vi "Change Unit.vi"(0 "Rigol DG822 Sine in":refnum<class "Rigol DG822 Sine.lvclass">, 9 "ParamTags":T1, 11 "error in (no error)":errorcluster, 12 "New Value":u16, 14 "Old Value":u16) -> (4 "Rigol DG822 Sine out":refnum<class "Rigol DG822 Sine.lvclass">, 15 "error out":errorcluster)   [LabVIEW 2021, in "Rigol DG822 UI.lvlib" / "Rigol DG822 Sine.lvlib" / "Rigol DG822 Sine.lvclass"]
uses:
  Rigol DG822 Sine.lvclass
  Rigol DG822 UI/lib/controls.llb/WaveformParamTags.ctl
  Rigol DG822 UI/lib/controls.llb/FreqUnit.ctl
  Rigol DG822 Sine.lvclass/Rigol DG822 Sine.ctl
  Rigol DG822 UI/lib/controls.llb/PeriodUnit.ctl
  Rigol DG822 UI/lib/controls.llb/AmplUnit.ctl
  Rigol DG822 UI/lib/controls.llb/HighLUnit.ctl
  Rigol DG822 UI/lib/controls.llb/OffsetUnit.ctl
  Rigol DG822 UI/lib/controls.llb/LowLUnit.ctl
  General/Files/lvlibp/Actors.lvlibp/Actors/Actors/Actors.lvclass
  D:/LabVIEW/General/Files/lvlibp/Actors.lvlibp/Actors/Actors/Actors.lvclass
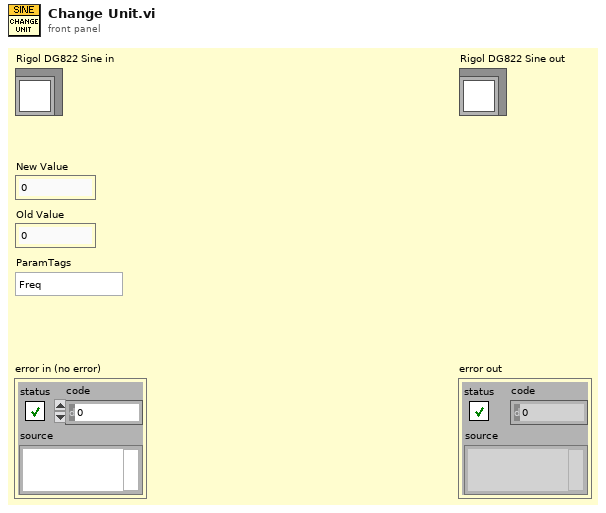
[diagram p1: front panel]
types:
  T1 = typedef "WaveformParamTags.ctl" = enum16{"Freq", "Period", "Ampl", "HighL", "Offset", "LowL", "Phase", "Duty", "Width", "RisEdge", "FallEdge"}
  T2 = typedef "FreqUnit.ctl" = enum32{"No Selection", "MHz", "kHz", "Hz", "mHz", "uHz"}
  T3 = typedef "PeriodUnit.ctl" = enum32{"No Selection", "s", "ms", "us", "ns"}
  T4 = typedef "AmplUnit.ctl" = enum32{"No Selection", "Vpp", "mVpp"}
  T5 = typedef "HighLUnit.ctl" = enum32{"No Selection", "V", "mV"}
  T6 = typedef "OffsetUnit.ctl" = enum32{"No Selection", "Vdc", "mVdc"}
  T7 = typedef "LowLUnit.ctl" = enum32{"No Selection", "V", "mV"}
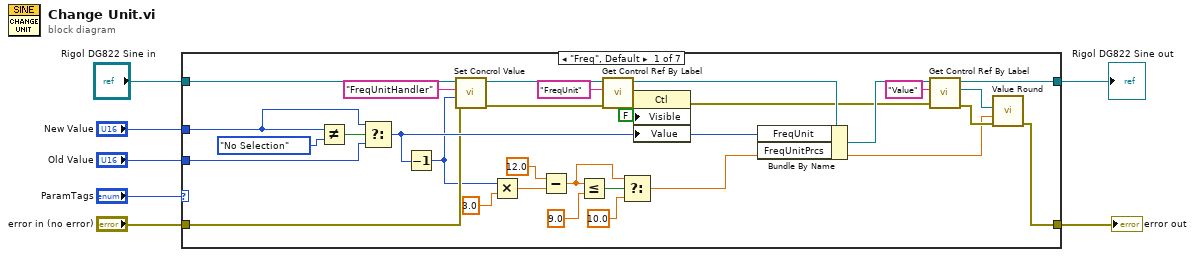
[diagram p0: block diagram]
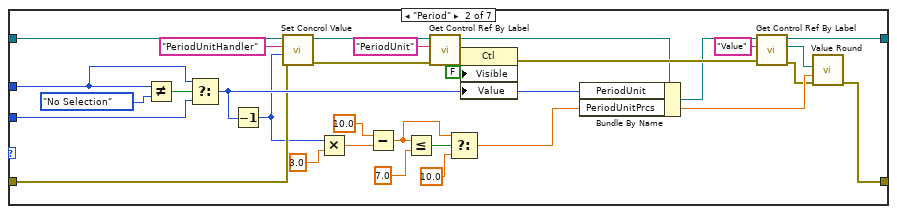
[diagram p2: hidden frame]
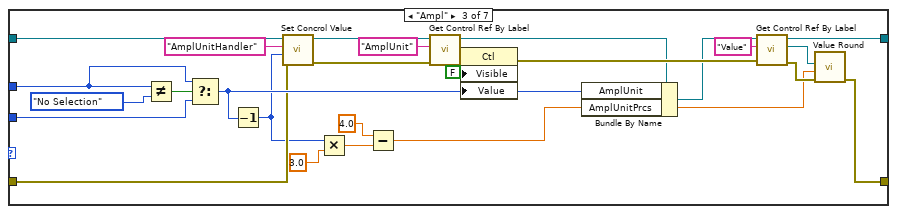
[diagram p3: hidden frame]
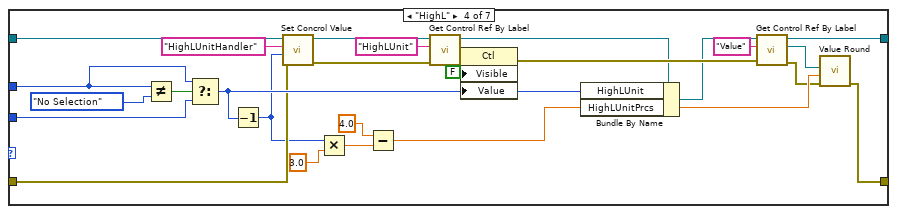
[diagram p4: hidden frame]
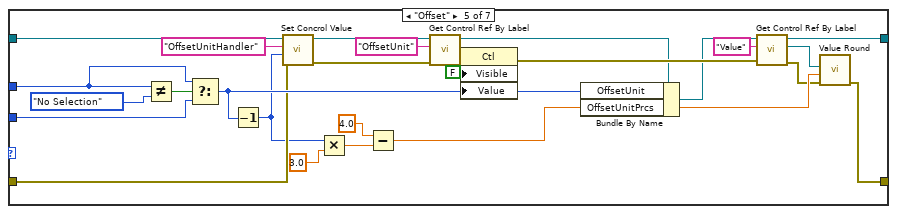
[diagram p5: hidden frame]
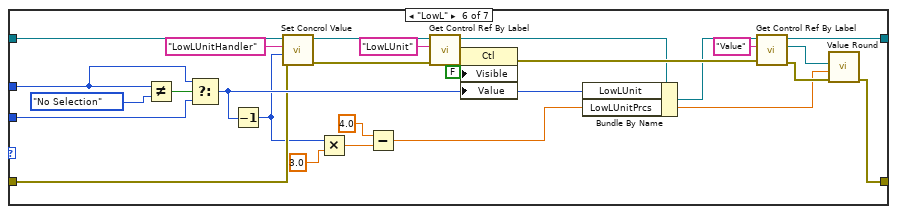
[diagram p6: hidden frame]
diagram:
  n1 = case shown="\"Freq\", Default" "ParamTags" {
    tunnel: [w8 w40 w70 w100 w124 w154 w179] -> w6
    tunnel: "error in (no error)" -> [w15 w48 w77 w104 w131 w158 w179]
    tunnel: [w14 w47 w76 w103 w130 w157 w178] -> w4
    tunnel: "Rigol DG822 Sine in" -> [w27 w57 w84 w111 w138 w165 w178]
    tunnel: "New Value" -> [w24 w55 w82 w109 w136 w163 _]
    tunnel: "Old Value" -> [w25 w56 w83 w110 w137 w164 _]
    frame "Freq", Default {
      n2 = Not Equal?(x=w24, y=FreqUnit."No Selection" ("x")) -> (x != y?=w35:bool)
      n3 = Select(t=w24, s=w35, f=w25) -> (s? t:f=w16:u16)
      n4 = Decrement(x=w16) -> (x-1=w13:u16)
      n5 = call "Set Concrol Value.vi"("error in (no error)"=w15, "Value"=w13, "Control Label"="FreqUnitHandler", "Actors in"=w27) -> ("error out"=w36:errorcluster, "Actors out"=w34:refnum<class "Rigol DG822 Sine.lvclass">)  [unwired: 6 in]
      n6 = Multiply(x=w13, y=3.0) -> (x*y=w21:dbl)
      n7 = Subtract(x=12.0, y=w21) -> (x-y=w23:dbl)
      n8 = Less Or Equal?(x=w23, y=9.0) -> (x <= y?=w22:bool)
      n9 = call "Get Control Ref By Label.vi"("error in (no error)"=w36, "Control Label"="FreqUnit", "Actors in"=w34) -> ("error out"=w37:errorcluster, "Control Ref"=w38:refnum<vi>, "Actors out"=w32:refnum<class "Rigol DG822 Sine.lvclass">)  [unwired: 6 in]
      n10 = Select(t=w23, s=w22, f=10.0 ("y")) -> (s? t:f=w10:dbl)
      n11 = property class="Ctl"(reference=w38, error in=w37, "Visible"=FALSE, "Value"=w16) -> (error out=w12:errorcluster)  [unwired: 1 out]
      n12 = Bundle By Name(cluster=w32, "FreqUnit"=w16, "FreqUnitPrcs"=w10) -> (w33:refnum<class "Rigol DG822 Sine.lvclass">)
      n13 = call "Get Control Ref By Label.vi"("error in (no error)"=w12, "Control Label"="Value", "Actors in"=w33) -> ("error out"=w11:errorcluster, "Control Ref"=w9:refnum<vi>, "Actors out"=w14:refnum<class "Rigol DG822 Sine.lvclass">)  [unwired: 6 in]
      n14 = call "Value Round.vi"("error in (no error)"=w11, "UnitPrecision"=w10, "Value Ref"=w9) -> ("error out"=w8:errorcluster)  [unwired: 7 in, 1 out]
    }
    frame "Period" {
      n15 = Not Equal?(x=w55, y=PeriodUnit."No Selection" ("x")) -> (x != y?=w66:bool)
      n16 = Select(t=w55, s=w66, f=w56) -> (s? t:f=w49:u16)
      n17 = Decrement(x=w49) -> (x-1=w46:u16)
      n18 = call "Set Concrol Value.vi"("error in (no error)"=w48, "Value"=w46, "Control Label"="PeriodUnitHandler", "Actors in"=w57) -> ("error out"=w67:errorcluster, "Actors out"=w65:refnum<class "Rigol DG822 Sine.lvclass">)  [unwired: 6 in]
      n19 = Multiply(x=w46, y=3.0) -> (x*y=w52:dbl)
      n20 = Subtract(x=10.0, y=w52) -> (x-y=w54:dbl)
      n21 = Less Or Equal?(x=w54, y=7.0) -> (x <= y?=w53:bool)
      n22 = call "Get Control Ref By Label.vi"("error in (no error)"=w67, "Control Label"="PeriodUnit", "Actors in"=w65) -> ("error out"=w68:errorcluster, "Control Ref"=w69:refnum<vi>, "Actors out"=w62:refnum<class "Rigol DG822 Sine.lvclass">)  [unwired: 6 in]
      n23 = Select(t=w54, s=w53, f=10.0 ("x")) -> (s? t:f=w43:dbl)
      n24 = property class="Ctl"(reference=w69, error in=w68, "Visible"=FALSE, "Value"=w49) -> (error out=w64:errorcluster)  [unwired: 1 out]
      n25 = Bundle By Name(cluster=w62, "PeriodUnit"=w49, "PeriodUnitPrcs"=w43) -> (w63:refnum<class "Rigol DG822 Sine.lvclass">)
      n26 = call "Get Control Ref By Label.vi"("error in (no error)"=w64, "Control Label"="Value", "Actors in"=w63) -> ("error out"=w41:errorcluster, "Control Ref"=w42:refnum<vi>, "Actors out"=w47:refnum<class "Rigol DG822 Sine.lvclass">)  [unwired: 6 in]
      n27 = call "Value Round.vi"("error in (no error)"=w41, "UnitPrecision"=w43, "Value Ref"=w42) -> ("error out"=w40:errorcluster)  [unwired: 7 in, 1 out]
    }
    frame "Ampl" {
      n28 = Not Equal?(x=w82, y=AmplUnit."No Selection" ("AmplUnit")) -> (x != y?=w93:bool)
      n29 = Select(t=w82, s=w93, f=w83) -> (s? t:f=w78:u16)
      n30 = Decrement(x=w78) -> (x-1=w75:u16)
      n31 = call "Set Concrol Value.vi"("error in (no error)"=w77, "Value"=w75, "Control Label"="AmplUnitHandler", "Actors in"=w84) -> ("error out"=w94:errorcluster, "Actors out"=w92:refnum<class "Rigol DG822 Sine.lvclass">)  [unwired: 6 in]
      n32 = Multiply(x=w75, y=3.0) -> (x*y=w81:dbl)
      n33 = Subtract(x=4.0, y=w81) -> (x-y=w71:dbl)
      n34 = call "Get Control Ref By Label.vi"("error in (no error)"=w94, "Control Label"="AmplUnit", "Actors in"=w92) -> ("error out"=w95:errorcluster, "Control Ref"=w96:refnum<vi>, "Actors out"=w89:refnum<class "Rigol DG822 Sine.lvclass">)  [unwired: 6 in]
      n35 = property class="Ctl"(reference=w96, error in=w95, "Visible"=FALSE, "Value"=w78) -> (error out=w91:errorcluster)  [unwired: 1 out]
      n36 = Bundle By Name(cluster=w89, "AmplUnit"=w78, "AmplUnitPrcs"=w71) -> (w90:refnum<class "Rigol DG822 Sine.lvclass">)
      n37 = call "Get Control Ref By Label.vi"("error in (no error)"=w91, "Control Label"="Value", "Actors in"=w90) -> ("error out"=w72:errorcluster, "Control Ref"=w73:refnum<vi>, "Actors out"=w76:refnum<class "Rigol DG822 Sine.lvclass">)  [unwired: 6 in]
      n38 = call "Value Round.vi"("error in (no error)"=w72, "UnitPrecision"=w71, "Value Ref"=w73) -> ("error out"=w70:errorcluster)  [unwired: 7 in, 1 out]
    }
    frame "HighL" {
      n39 = Not Equal?(x=w109, y=HighLUnit."No Selection" ("HighLUnit")) -> (x != y?=w120:bool)
      n40 = Select(t=w109, s=w120, f=w110) -> (s? t:f=w105:u16)
      n41 = Decrement(x=w105) -> (x-1=w102:u16)
      n42 = call "Set Concrol Value.vi"("error in (no error)"=w104, "Value"=w102, "Control Label"="HighLUnitHandler", "Actors in"=w111) -> ("error out"=w121:errorcluster, "Actors out"=w119:refnum<class "Rigol DG822 Sine.lvclass">)  [unwired: 6 in]
      n43 = Multiply(x=w102, y=3.0) -> (x*y=w108:dbl)
      n44 = Subtract(x=4.0, y=w108) -> (x-y=w99:dbl)
      n45 = call "Get Control Ref By Label.vi"("error in (no error)"=w121, "Control Label"="HighLUnit", "Actors in"=w119) -> ("error out"=w122:errorcluster, "Control Ref"=w123:refnum<vi>, "Actors out"=w116:refnum<class "Rigol DG822 Sine.lvclass">)  [unwired: 6 in]
      n46 = property class="Ctl"(reference=w123, error in=w122, "Visible"=FALSE, "Value"=w105) -> (error out=w118:errorcluster)  [unwired: 1 out]
      n47 = Bundle By Name(cluster=w116, "HighLUnit"=w105, "HighLUnitPrcs"=w99) -> (w117:refnum<class "Rigol DG822 Sine.lvclass">)
      n48 = call "Get Control Ref By Label.vi"("error in (no error)"=w118, "Control Label"="Value", "Actors in"=w117) -> ("error out"=w98:errorcluster, "Control Ref"=w97:refnum<vi>, "Actors out"=w103:refnum<class "Rigol DG822 Sine.lvclass">)  [unwired: 6 in]
      n49 = call "Value Round.vi"("error in (no error)"=w98, "UnitPrecision"=w99, "Value Ref"=w97) -> ("error out"=w100:errorcluster)  [unwired: 7 in, 1 out]
    }
    frame "Offset" {
      n50 = Not Equal?(x=w136, y=OffsetUnit."No Selection" ("OffsetUnit")) -> (x != y?=w147:bool)
      n51 = Select(t=w136, s=w147, f=w137) -> (s? t:f=w132:u16)
      n52 = Decrement(x=w132) -> (x-1=w129:u16)
      n53 = call "Set Concrol Value.vi"("error in (no error)"=w131, "Value"=w129, "Control Label"="OffsetUnitHandler", "Actors in"=w138) -> ("error out"=w148:errorcluster, "Actors out"=w146:refnum<class "Rigol DG822 Sine.lvclass">)  [unwired: 6 in]
      n54 = Multiply(x=w129, y=3.0) -> (x*y=w135:dbl)
      n55 = Subtract(x=4.0, y=w135) -> (x-y=w127:dbl)
      n56 = call "Get Control Ref By Label.vi"("error in (no error)"=w148, "Control Label"="OffsetUnit", "Actors in"=w146) -> ("error out"=w149:errorcluster, "Control Ref"=w150:refnum<vi>, "Actors out"=w143:refnum<class "Rigol DG822 Sine.lvclass">)  [unwired: 6 in]
      n57 = property class="Ctl"(reference=w150, error in=w149, "Visible"=FALSE, "Value"=w132) -> (error out=w145:errorcluster)  [unwired: 1 out]
      n58 = Bundle By Name(cluster=w143, "OffsetUnit"=w132, "OffsetUnitPrcs"=w127) -> (w144:refnum<class "Rigol DG822 Sine.lvclass">)
      n59 = call "Get Control Ref By Label.vi"("error in (no error)"=w145, "Control Label"="Value", "Actors in"=w144) -> ("error out"=w125:errorcluster, "Control Ref"=w126:refnum<vi>, "Actors out"=w130:refnum<class "Rigol DG822 Sine.lvclass">)  [unwired: 6 in]
      n60 = call "Value Round.vi"("error in (no error)"=w125, "UnitPrecision"=w127, "Value Ref"=w126) -> ("error out"=w124:errorcluster)  [unwired: 7 in, 1 out]
    }
    frame "LowL" {
      n61 = Not Equal?(x=w163, y=LowLUnit."No Selection" ("LowLUnit")) -> (x != y?=w174:bool)
      n62 = Select(t=w163, s=w174, f=w164) -> (s? t:f=w159:u16)
      n63 = Decrement(x=w159) -> (x-1=w156:u16)
      n64 = call "Set Concrol Value.vi"("error in (no error)"=w158, "Value"=w156, "Control Label"="LowLUnitHandler", "Actors in"=w165) -> ("error out"=w175:errorcluster, "Actors out"=w173:refnum<class "Rigol DG822 Sine.lvclass">)  [unwired: 6 in]
      n65 = Multiply(x=w156, y=3.0) -> (x*y=w162:dbl)
      n66 = Subtract(x=4.0, y=w162) -> (x-y=w152:dbl)
      n67 = call "Get Control Ref By Label.vi"("error in (no error)"=w175, "Control Label"="LowLUnit", "Actors in"=w173) -> ("error out"=w176:errorcluster, "Control Ref"=w177:refnum<vi>, "Actors out"=w170:refnum<class "Rigol DG822 Sine.lvclass">)  [unwired: 6 in]
      n68 = property class="Ctl"(reference=w177, error in=w176, "Visible"=FALSE, "Value"=w159) -> (error out=w172:errorcluster)  [unwired: 1 out]
      n69 = Bundle By Name(cluster=w170, "LowLUnit"=w159, "LowLUnitPrcs"=w152) -> (w171:refnum<class "Rigol DG822 Sine.lvclass">)
      n70 = call "Get Control Ref By Label.vi"("error in (no error)"=w172, "Control Label"="Value", "Actors in"=w171) -> ("error out"=w153:errorcluster, "Control Ref"=w151:refnum<vi>, "Actors out"=w157:refnum<class "Rigol DG822 Sine.lvclass">)  [unwired: 6 in]
      n71 = call "Value Round.vi"("error in (no error)"=w153, "UnitPrecision"=w152, "Value Ref"=w151) -> ("error out"=w154:errorcluster)  [unwired: 7 in, 1 out]
    }
    frame "Phase" {
    }
  }
  "error out" <- w6
  "Rigol DG822 Sine out" <- w4
